vi "getShutterStatus.vi"(6 "Delay between send and receive [ms]":i32=100, 8 "error in (no error)":errorcluster, 11 "Monochromator in":refnum<class "Monochromator.lvclass">) -> (0 "error out":errorcluster, 1 "Shutter 2":i32, 2 "Shutter 1":i32, 3 "Monochromator out":refnum<class "Monochromator.lvclass">)   [LabVIEW 2023, in "Monochromator.lvclass"]
uses:
  Monochromator.lvclass
  Monochromator.lvclass/Monochromator.ctl
  d9b87029-586e-44ee-a6e5-d4a5e0edce38.vi
  b59fd1e7-dcda-425c-bd6c-61aafb79e7f4.vi
  GenericDevice/GenericDevice.lvclass
  <vilib>/IlluminatedG/lv-web-crypto/lv-json/JSON/JSON.lvlib
  ShutterStatus.ctl
panel:
  # "Connector Pane"
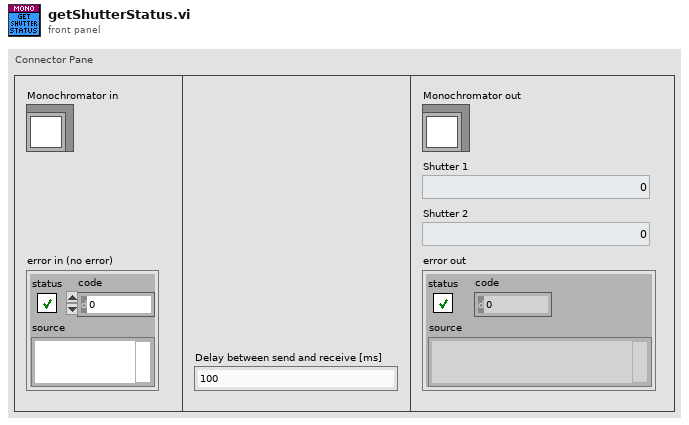
[diagram p1: front panel]
types:
  T1 = typedef "Monochromator.lvclass/ShutterStatus.ctl" = cluster{"Shutter 1":i32, "Shutter 2":i32}
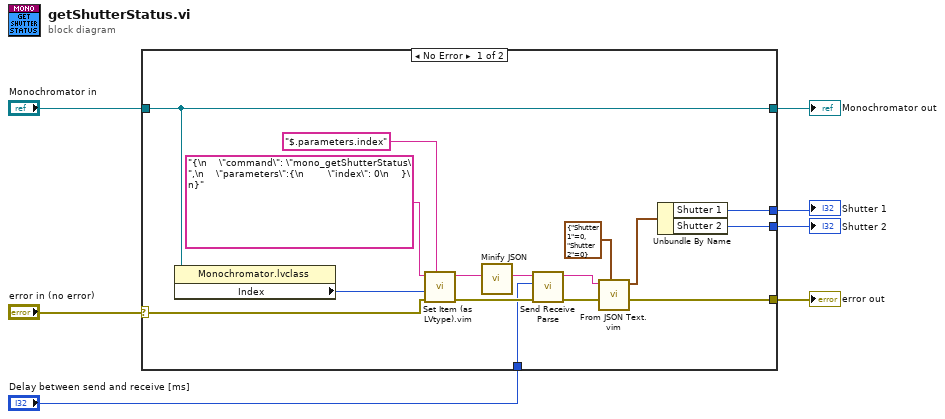
[diagram p0: block diagram]
diagram:
  n1 = case shown="No Error" "error in (no error)" {
    selector: "error in (no error)" -> [w19 w25]
    tunnel: [w18 w25] -> w6
    tunnel: [w21 w24] -> w4
    tunnel: "Monochromator in" -> [w21 w24]
    tunnel: [w10 _] -> w3
    tunnel: [w9 _] -> w2
    tunnel: "Delay between send and receive [ms]" -> [w8 _]
    frame No Error {
      n2 = property class="Monochromator.lvclass"(reference=w21) -> ("Index"=w20:i32)  [unwired: 1 in, 2 out]
      n3 = call "Set Item (as LVtype).vim"("$Path or Item Name"="$.parameters.index", "error in (no error)"=w19, "Anything"=w20, "JSON"="{\n    \"command\": \"mono_getShutterStatus\",\n    \"parameters\":{\n        \"index\": 0\n    }\n}") -> ("error out"=w17:errorcluster, "<JSON>"=w14:string)  [unwired: 4 in, 1 out]
      n4 = call <vilib>:"Minify JSON.vi"("JSON String"=w14) -> ("Minified JSON"=w13:string)  [unwired: 10 in]
      n5 = call "Send Receive Parse.vi"("error in"=w17, "Delay between send and receive [ms]"=w8, "<JSON>"=w13) -> ("error out"=w15:errorcluster, "results-JSON string"=w16:string)  [unwired: 6 in, 1 out]
      n6 = call "From JSON Text.vim"("Data Type and Default Value"=T1 {"Shutter 1"=0, "Shutter 2"=0} ("Selected Shutter"), "error in (no error)"=w15, "JSON"=w16) -> ("error out"=w18:errorcluster, "Data out"=w12:T1)  [unwired: 7 in]
      n7 = Unbundle By Name(w12) -> ("Shutter 1"=w10:i32, "Shutter 2"=w9:i32)
    }
    frame Error {
    }
  }
  "error out" <- w6
  "Monochromator out" <- w4
  "Shutter 1" <- w3
  "Shutter 2" <- w2
